vi "BNC555.Initialize.vi"(0 "i ref in":refnum<vi>, 1 "Id Query (true)":bool caption="id query (false)", 2 "Reset (true)":bool caption="reset device (false)", 5 "error in (no error)":errorcluster) -> (14 "i ref out":refnum<vi>, 19 "error out":errorcluster)   [LabVIEW 2014, in "BNC555.lvlib"]
doc: "This VI initializes the connection to the hardare and sets several GUI elements."
uses:
  BNC555.lvlib
  non_GPL/instr.lib/BNC555/BNC555 - Driver np.lvlib
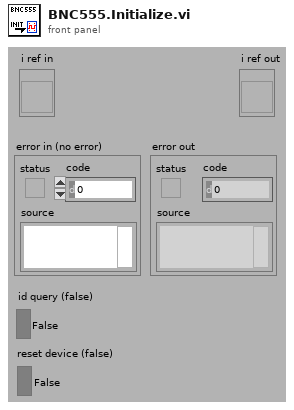
[diagram p1: front panel]
types:
  T1 = typedef "BNC555.lvlib/BNC555.i attribute.ctl" = cluster{"Information":cluster{"VISA resource name":refnum<visa-resource-name>, "Baud Rate (1:9600)":u16}, "Channel Array":T2[], "System":T3, "GUI Refs":cluster{"Delete":refnum<vi>, "Information":refnum<vi>, "System":refnum<vi>, "Channel Array":refnum<vi>, "Device Error":refnum<vi>, "Instr Driver Revision":refnum<vi>, "Instr Firmware Revision":refnum<vi>, "Instr Option":refnum<vi>, "Self-Test Response":refnum<vi>}, "Service IDs Channelinfo":i32[], "Service ID T0 Mode":i32}
  T2 = typedef "BNC555 - Driver np.lvlib/BNC555 All Chan Parameters.ctl" = cluster{"Chan #":i32, "Chan State":bool, "Chan Delay":dbl, "Chan Width":dbl, "Chan Mode":enum16{"Normal", "Single", "Burst", "Divide by N"}, "Chan Burst #":u32, "Chan Divide #":u32, "Chan Pol Out":enum16{"Normal", "Complement", "Inverted"}, "Chan Level Out":enum16{"TTL", "Adjustable", "35 Volt"}, "Chan Lev Adjust":dbl, "Chan Gate Pol":enum16{"Normal", "Complement", "Inverted"}, "Chan Gate State":bool}
  T3 = typedef "BNC555 - Driver np.lvlib/BNC555 All Sys Parameters.ctl" = cluster{"Sys Period":dbl, "Sys Oscillator":bool, "Sys Mode":enum16{"Normal", "Single", "Burst", "Duty Cycle"}, "Sys Burst #":u32, "Sys DC On":u32, "Sys DC Off":u32, "Sys Trig Mode":enum16{"Disabled", "Triggered", "Gated"}, "Sys Trig Lev":dbl, "Sys Gate State":bool, "Sys Trig Edge":bool, "Sys State":bool}
  T4 = cluster{"VISA resource name":refnum<visa-resource-name>, "Baud Rate (1:9600)":u16}
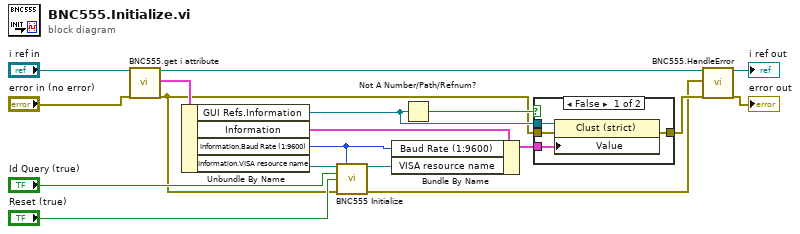
[diagram p0: block diagram]
diagram:
  n1 = call "BNC555.get i attribute.vi"("i ref in"="i ref in", "error in (no error)"="error in (no error)") -> ("i ref out"=w4:refnum<vi>, "i attribute"=w16:T1, "error out"=w9:errorcluster)  [unwired: 15 in]
  n2 = Unbundle By Name(w16) -> ("GUI Refs.Information"=w10:refnum<vi>, "Information"=w2:T4, "Information.Baud Rate (1:9600)"=w6:u16, "Information.VISA resource name"=w13:refnum<visa-resource-name>)
  n3 = call "BNC555 Initialize.vi"("VISA resource"=w13, "Baud Rate (1:9600)"=w6, "ID Query (T: Check)"="Id Query (true)", "Reset (T: Reset)"="Reset (true)", "error in (no error)"=w9) -> ("dup VISA resource"=w7:refnum<visa-resource-name>, "error out"=w1:errorcluster)  [unwired: 9 in]
  n4 = Bundle By Name(cluster=w2, "Baud Rate (1:9600)"=w6, "VISA resource name"=w7) -> (w8:T4)
  n5 = Not A Number/Path/Refnum?(number/path/refnum=w10) -> (NaN/Path/Refnum?=w11:bool)
  n6 = case shown="False" w11 {
    tunnel: w9 -> [w22 w23]
    tunnel: [w21 w23] -> w5
    tunnel: w10 -> [w20 _]
    tunnel: w8 -> [w19 _]
    frame False {
      n7 = property class="Clust (strict)"(reference=w20, error in=w22, "Value"=w19) -> (error out=w21:errorcluster)  [unwired: 1 out]
    }
    frame True {
    }
  }
  n8 = call "BNC555.HandleError.vi"("i ref in"=w4, "Device error"=w1, "error in (no error)"=w5) -> ("i ref out"=→"i ref out":refnum<vi>, "error out"=→"error out":errorcluster)  [unwired: 15 in]
